vi "data_transform subVI.vi"(0 "data":dbl[][](array[numeric]), 11 "error in (no error)":errorcluster) -> (4 "Array":dbl[](array[numeric]), 15 "error out":errorcluster)   [LabVIEW 2018]
uses:
  <vilib>/Analysis/2dsp.llb/Real FFT.vi
  <vilib>/Analysis/5stat.llb/RMS (DBL).vi
  <vilib>/Analysis/NI_AALBase.lvlib
  <vilib>/Analysis/NI_AALPro.lvlib
  <vilib>/gmath/NI_Gmath.lvlib
panel:
  out "output array":dbl[](array[numeric])
  out "Array 2":dbl[][](array[numeric])
  out "kurtosis":dbl[](array[numeric])
  out "skewness":dbl[](array[numeric])
  out "rms value":dbl[](array[numeric]) format="%0.2f"
  out "variance":dbl[](array[numeric]) format="%0.2f"
  out "standard deviation":dbl[](array[numeric]) format="%0.2f"
  out "mean":dbl[](array[numeric]) format="%0.2f"
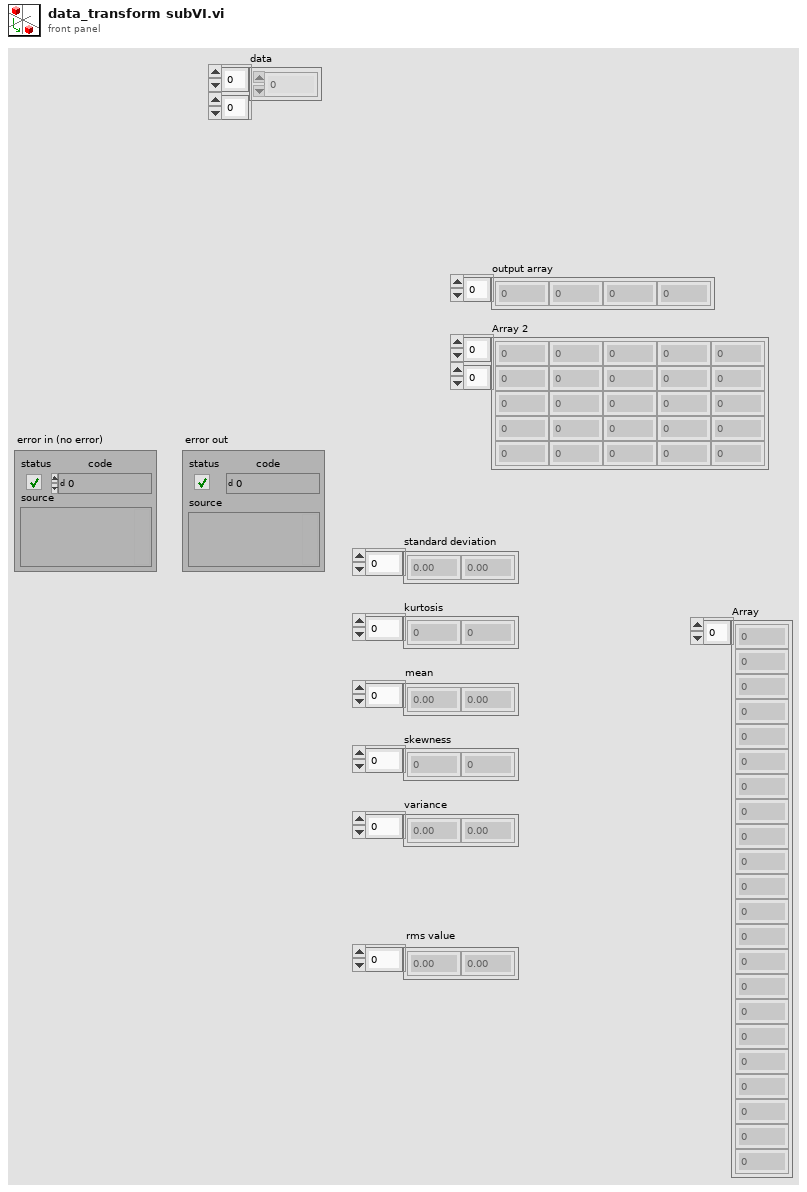
[diagram p1: front panel]
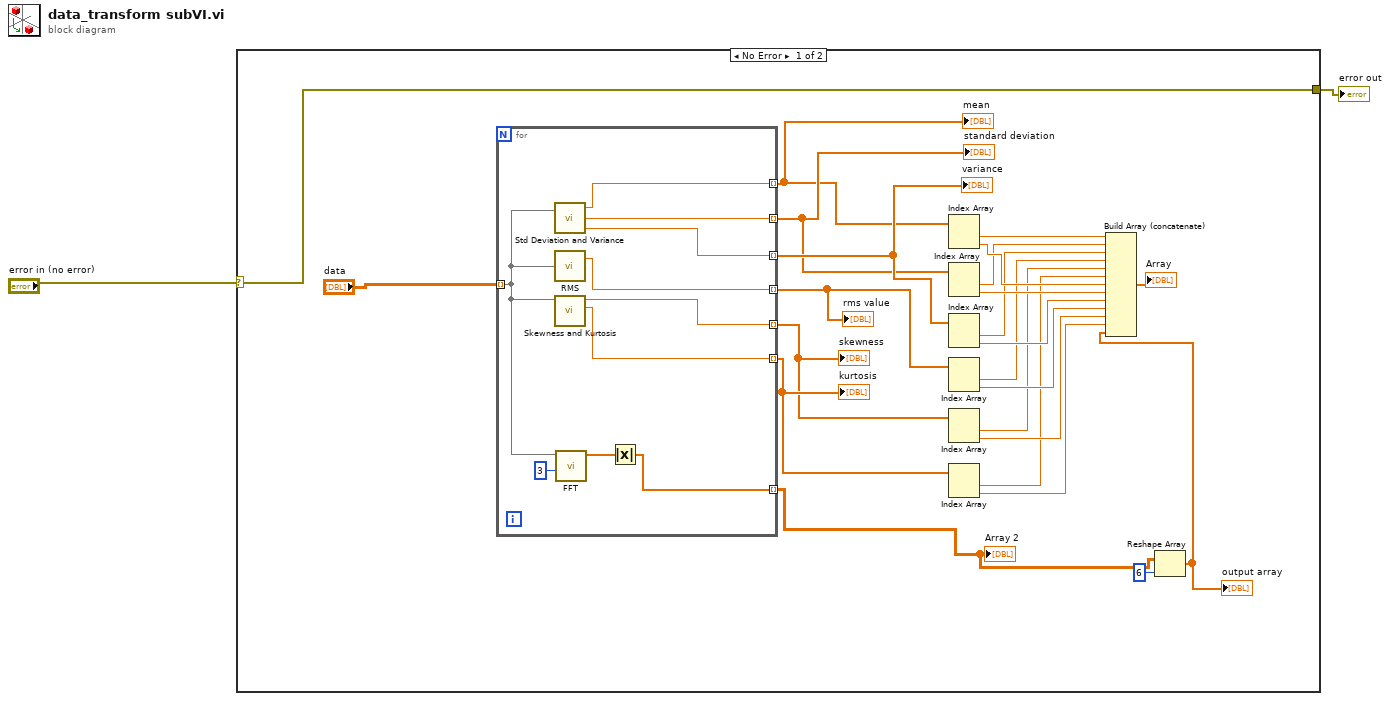
[diagram p0: block diagram]
diagram:
  n1 = case shown="No Error" "error in (no error)" {
    selector: "error in (no error)" -> [w6 w37]
    tunnel: [w6 w37] -> w1
    frame No Error {
      n2 = for {
        tunnel: "data" -> [w28] mode=indexing
        tunnel: [w36] -> w17 mode=indexing
        tunnel: [w35] -> w16 mode=indexing
        tunnel: [w34] -> w15 mode=indexing
        tunnel: [w33] -> w12 mode=indexing
        tunnel: [w32] -> w10 mode=indexing
        tunnel: [w31] -> w8 mode=indexing
        tunnel: [w27] -> w5 mode=indexing
        n3 = call <vilib>:"Std Deviation and Variance.vi"("X"=w28) -> ("mean"=w31:dbl, "standard deviation"=w32:dbl, "variance"=w33:dbl)  [unwired: 1 in]
        n4 = call-poly <vilib>:"RMS.vi"("X"=w28) -> ("rms value"=w34:dbl)  [unwired: 1 out]
        n5 = call <vilib>:"Skewness and Kurtosis.vi"("X"=w28) -> ("kurtosis"=w36:dbl, "skewness"=w35:dbl)  [unwired: 8 in, 1 out]
        n6 = call-poly <vilib>:"FFT.vi"("FFT size"=3, "X"=w28) -> ("FFT {X}"=w29:cdb[])  [unwired: 8 in, 1 out]
        n7 = Absolute Value(x=w29) -> (abs(x)=w27:dbl[])
      }
      "mean" <- w8
      "standard deviation" <- w10
      "variance" <- w12
      "rms value" <- w15
      "skewness" <- w16
      "kurtosis" <- w17
      "Array 2" <- w5
      n8 = Index Array(array=w8) -> (element #1=w9:dbl, element #2=w20:dbl)  [unwired: 2 in]
      n9 = Index Array(array=w10) -> (element #1=w11:dbl, element #2=w21:dbl)  [unwired: 2 in]
      n10 = Index Array(array=w12) -> (element #1=w13:dbl, element #2=w22:dbl)  [unwired: 2 in]
      n11 = Index Array(array=w15) -> (element #1=w14:dbl, element #2=w23:dbl)  [unwired: 2 in]
      n12 = Index Array(array=w16) -> (element #1=w18:dbl, element #2=w24:dbl)  [unwired: 2 in]
      n13 = Index Array(array=w17) -> (element #1=w19:dbl, element #2=w25:dbl)  [unwired: 2 in]
      n14 = Reshape Array(w5, 6 ("dimension size")) -> (w4:dbl[])
      "output array" <- w4
      n15 = Build Array (concatenate)(w9, w11, w13, w14, w18, w19, w20, w21, w22, w23, w24, w25, w4) -> (→"Array":dbl[])
    }
    frame Error {
    }
  }
  "error out" <- w1
